vi "Get latest RSS and all addons.vi"(8 "error in (no error)":errorcluster, 10 "Repository Location":string, 11 "RT Management in":refnum<class "RT Management.lvclass">) -> (0 "error out":errorcluster, 1 "add-ons":T1[](array[typedef]) {"component type" items=["standard", "hidden", "system", "unknown", "startup", "image"]}, 2 "software set":T1 {"component type" items=["standard", "hidden", "system", "unknown", "startup", "image"]}, 3 "RT Management out":refnum<class "RT Management.lvclass">, 4 "items":T1[](array[typedef]) {"component type" items=["standard", "hidden", "system", "unknown", "startup", "image"]})   [LabVIEW 2016, in "RT Management.lvlib" / "RT Management.lvclass"]
uses:
  RT Management.lvclass
  <vilib>/nisyscfg/Software 1.2.ctl
  <vilib>/nisyscfg/Component Type.ctl
  <vilib>/nisyscfg/Component Types.ctl
  RT Management.lvclass/RT Management.ctl
  Get SysCfg Session.vi
  <vilib>/nisyscfg/Get Available Sets.vi
  <vilib>/nisyscfg/Get Filtered Sets.vi
  <resource>/objmgr/nisysapi.rc
  <vilib>/nisyscfg/nisyscfg.lvlib
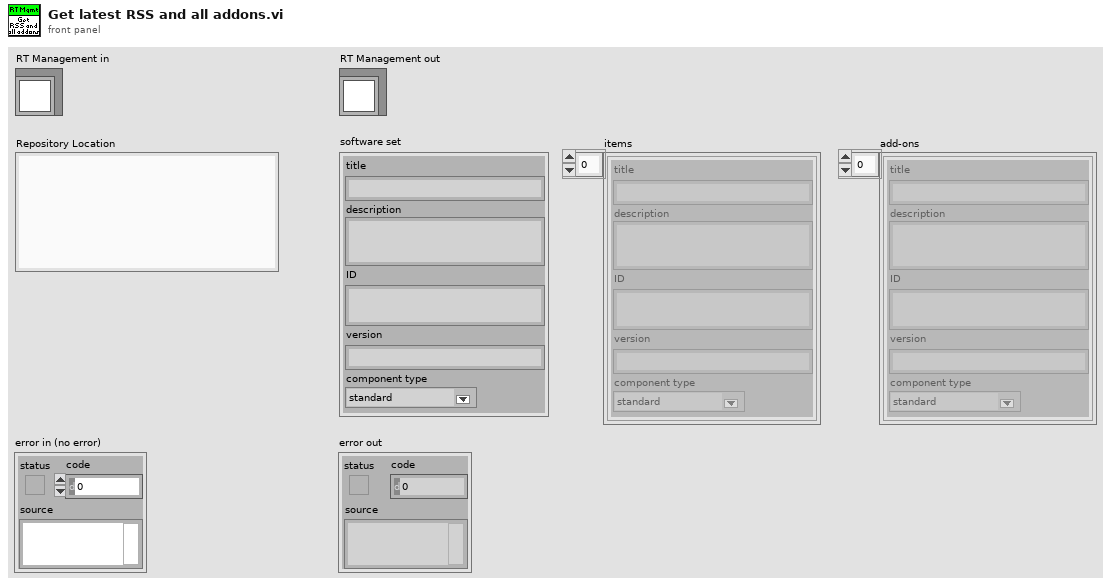
[diagram p1: front panel]
types:
  T1 = typedef "nisyscfg.lvlib/Software 1.2.ctl" = cluster{"title":string, "description":string, "ID":string, "version":string, "component type":T2}
  T2 = typedef "nisyscfg.lvlib/Component Type.ctl" = u32
  T3 = typedef "nisyscfg.lvlib/Component Types.ctl" = u32
  T4 = typedef "nisyscfg.lvlib/Software Set 1.2.ctl" = cluster{"information":T1, "items":T1[], "add-ons":T1[]}
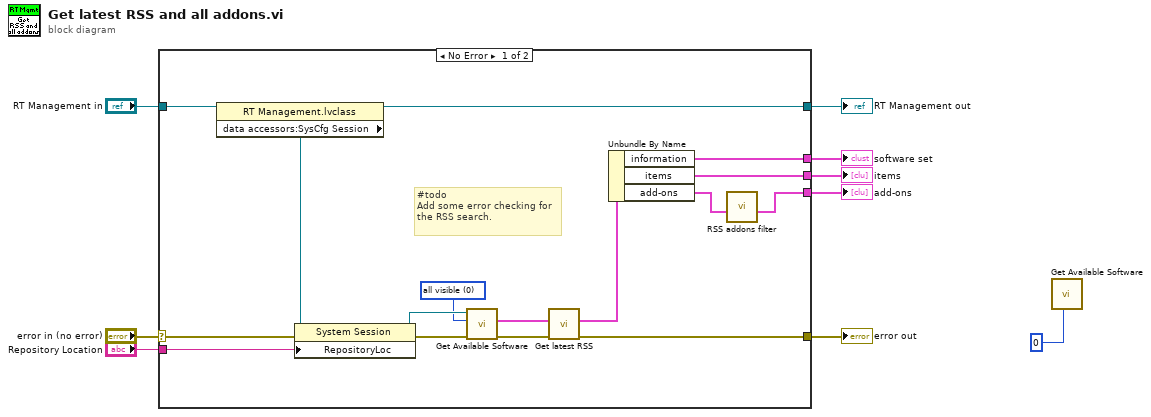
[diagram p0: block diagram]
diagram:
  n1 = case shown="No Error" "error in (no error)" {
    selector: "error in (no error)" -> [w25 w27]
    tunnel: [w14 w27] -> w8
    tunnel: [w22 w26] -> w6
    tunnel: "RT Management in" -> [w24 w26]
    tunnel: "Repository Location" -> [w19 _]
    tunnel: [w15 _] -> w4
    tunnel: [w17 _] -> w3
    tunnel: [w16 _] -> w2
    frame No Error {
      w18 = T3 0 items=["all visible", "all including hidden", "standard only", "startup only"] ("item types (visible)")
      # "#todo\nAdd some error checking for the RSS search."
      n2 = property class="RT Management.lvclass"(reference=w24) -> (reference out=w22:refnum<class "RT Management.lvclass">, "data accessors:SysCfg Session"=w23:refnum<k21>)  [unwired: 1 in, 1 out]
      n3 = property class="System Session"(reference=w23, error in=w25, "RepositoryLoc"=w19) -> (reference out=w20:refnum<k21>, error out=w21:errorcluster)
      n4 = call-poly <vilib>:"Get Available Software.vi"("error in (no error)"=w21, "Item Types (all visible)"=w18, "Session in"=w20) -> ("error out"=w13:errorcluster, "Software Sets"=w12:T4[])  [unwired: 6 in, 1 out]
      n5 = call "Get latest RSS.vi"("error in (no error)"=w13, "software sets"=w12) -> ("error out"=w14:errorcluster, "software set"=w11:T4)  [unwired: 8 in]
      n6 = Unbundle By Name(w11) -> ("information"=w16:T1, "items"=w15:T1[], "add-ons"=w10:T1[])
      n7 = call "RSS addons filter.vi"("add-ons"=w10) -> ("add-ons out"=w17:T1[])  [unwired: 10 in]
    }
    frame Error {
    }
  }
  "error out" <- w8
  "RT Management out" <- w6
  "items" <- w4
  "add-ons" <- w3
  "software set" <- w2
  n8 = call-poly <vilib>:"Get Available Software.vi"("Product ID"=0) -> ()  [unwired: 8 in, 3 out]
